vi "TCP - Client.vi"() -> ()   [LabVIEW 2020]
doc: "Demonstrates how to set up a basic TCP connection, send data to the specified port once a connection has been established, and terminate the connection once the data has been sent. This VI is designed to stop if the TCP connection is terminated. The data sent in this example is an array of random numbers."
panel:
  in  "Input string":string
  in  "Server Closed":string="The server VI closed the connection."
  in  "Stop":bool
  # "Slanje funkcionise tako sto se sanje broj releja, \na zati 0/1 u zavisnosti da li zelimo da ga ukljucimo ili iskljucimo."
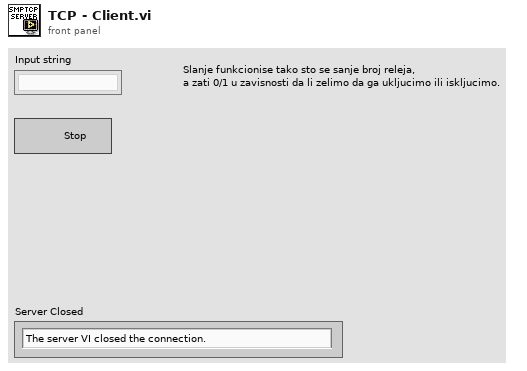
[diagram p1: front panel]
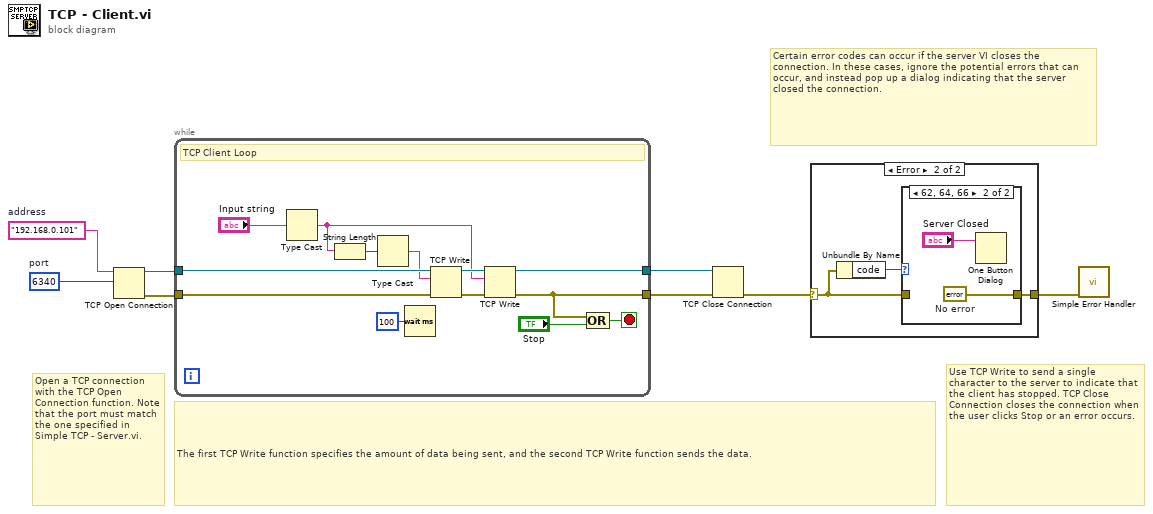
[diagram p0: block diagram]
diagram:
  w7 = u16 6340  # port
  w8 = "192.168.0.101"  # address
  # "Use TCP Write to send a single character to the server to indicate that the client has stopped. TCP Close Connection closes the connection when the user clicks Stop or an error occurs."
  # "Certain error codes can occur if the server VI closes the connection. In these cases, ignore the potential errors that can occur, and instead pop up a dialog indicating that the server closed the connection."
  # "Open a TCP connection with the TCP Open Connection function. Note that the port must match the one specified in Simple TCP - Server.vi."
  # "The first TCP Write function specifies the amount of data being sent, and the second TCP Write function sends the data."
  n1 = TCP Open Connection(address=w8, remote port or service name=w7) -> (connection ID=w6:refnum<k5>, error out=w5:errorcluster)  [unwired: 3 in]
  n2 = while {
    tunnel: [w10] -> w1
    tunnel: [w11] -> w2
    tunnel: w6 -> [w21]
    tunnel: w5 -> [w13]
    stop <- w14 stop-if-true
    # "TCP Client Loop"
    n3 = Type Cast(x="Input string") -> (*(type *) &x=w16:string)  [unwired: 1 out]
    n4 = String Length(string=w16) -> (length=w18:i32)
    n5 = Type Cast(x=w18) -> (*(type *) &x=w17:string)  [unwired: 1 out]
    n6 = Wait (ms)(milliseconds to wait=u32 100) -> ()  [unwired: 1 out]
    n7 = TCP Write(connection ID=w21, data in=w17, error in (no error)=w13) -> (connection ID out=w20:refnum<k5>, error out=w19:errorcluster)  [unwired: 2 out]
    n8 = TCP Write(connection ID=w20, data in=w16, error in (no error)=w19) -> (connection ID out=w11:refnum<k5>, error out=w10:errorcluster)  [unwired: 2 out]
    n9 = Compound Arithmetic op=OR(w10, "Stop") -> (w14:bool)
  }
  n10 = TCP Close Connection(connection ID=w2, error in (no error)=w1) -> (error out=w4:errorcluster)  [unwired: 1 in, 1 out]
  n11 = case shown="Error" w4 {
    selector: w4 -> [w22 w24]
    tunnel: [w22 w23] -> w3
    frame No Error {
    }
    frame Error {
      n12 = Unbundle By Name(w24) -> ("code"=w25:i32)
      n13 = case shown="62, 64, 66" w25 {
        tunnel: w24 -> [w26 _]
        tunnel: [w26 w28] -> w23
        frame Default {
        }
        frame 62, 64, 66 {
          w28 = errorcluster {"status"=FALSE, "code"=0, "source"=""}  # No error
          n14 = One Button Dialog(message="Server Closed") -> ()  [unwired: 1 in, 1 out]
        }
      }
    }
  }
  n15 = call <vilib>:"Simple Error Handler.vi"("error in (no error)"=w3) -> ()  [unwired: 4 in, 5 out]
